vi "Marker to Point Array.vi"(8 "error in (no error)":errorcluster, 11 "Overlay Ref":refnum<k24>) -> (0 "error out":errorcluster, 3 "Point Array":refnum<k24>)   [LabVIEW 2014]
uses:
  C:/Robotic Systems/Products/AgFalcon/Software/Ground Station/Data/Mapping DLL/GMap.NET.WindowsForms.dll
  Data/Mapping DLL/GMap.NET.WindowsForms.dll
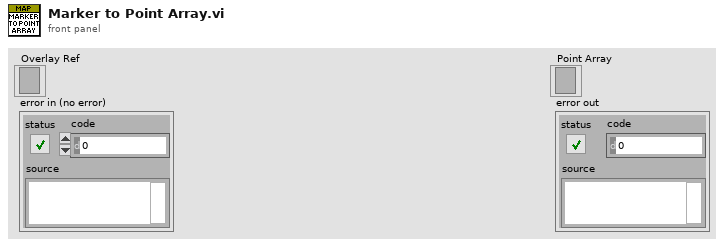
[diagram p1: front panel]
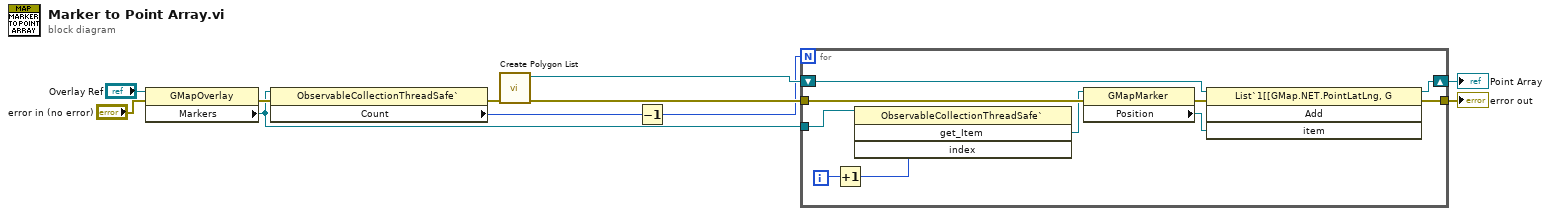
[diagram p0: block diagram]
diagram:
  n1 = property class="GMapOverlay"(reference="Overlay Ref", error in="error in (no error)") -> (error out=w11:errorcluster, "Markers"=w10:refnum<k24>)  [unwired: 1 out]
  n2 = property class="ObservableCollectionThreadSafe`"(reference=w10, error in=w11) -> (error out=w8:errorcluster, "Count"=w2:i32)  [unwired: 1 out]
  n3 = call "Create Polygon List.vi"("error in (no error)"=w8) -> ("error out"=w7:errorcluster, "specific class reference"=w9:refnum<k24>)  [unwired: 9 in]
  n4 = Decrement(x=w2) -> (x-1=w1:i32)
  n5 = for {
    N: w1 -> [_]
    tunnel: w7 -> [w18]
    shift-right: [w19] -> w6
    shift-left: w9 -> [w21]
    tunnel: [w16] -> w3
    tunnel: w10 -> [w15]
    i -> [w13]
    n6 = Increment(x=w13) -> (x+1=w12:i32)
    n7 = invoke class="ObservableCollectionThreadSafe`" method="get_Item"(reference=w15, "index"=w12) -> ("get_Item"=w14:refnum<k24>)  [unwired: 2 in, 3 out]
    n8 = property class="GMapMarker"(reference=w14, error in=w18) -> (error out=w17:errorcluster, "Position"=w20:refnum<k24>)  [unwired: 1 out]
    n9 = invoke class="List`1[[GMap.NET.PointLatLng, G" method="Add"(reference=w21, error in=w17, "item"=w20) -> (reference out=w19:refnum<k24>, error out=w16:errorcluster)  [unwired: 1 in, 2 out]
  }
  "Point Array" <- w6
  "error out" <- w3
